vi "testRegEvtServersAandB.vi"(8 "error in (no error)":errorcluster) -> (0 "error out":errorcluster)   [LabVIEW 2018]
uses:
  src/FactoryTcpServer/FactoryTcpServer.lvclass
  src/TcpServer/TcpServer.lvclass/TcpServer.ctl
  src/TcpServerBase/TcpServerBase.lvclass/TcpServerBase.ctl
  src/TcpServerCmd/TcpServerCmd.lvclass
  home/pcortes/Documents/github/ts_labview_tcp_json/src/TcpServerBase/TcpServerBase.lvclass
  <vilib>/addons/_JKI Toolkits/Caraya/classes/Assert/Assert Equal Value_Variant.vi
  <vilib>/addons/_JKI Toolkits/Caraya/classes/Test/Test.lvclass
  <vilib>/addons/_JKI Toolkits/Caraya/classes/Assert/Assert.lvclass
  src/TcpServer/TcpServer.lvclass
  src/TcpServerBase/TcpServerBase.lvclass
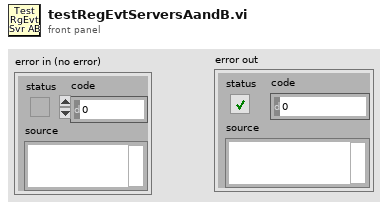
[diagram p1: front panel]
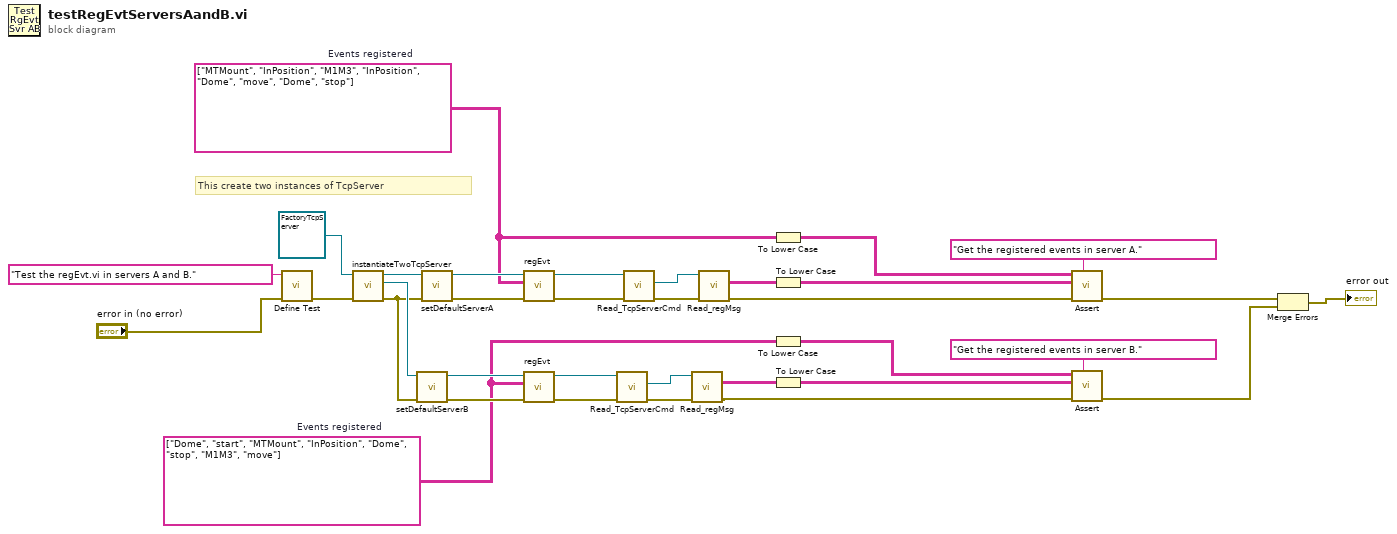
[diagram p0: block diagram]
diagram:
  w8 = string[][] [["Dome", "start"], ["MTMount", "InPosition"], ["Dome", "stop"], ["M1M3", "move"]]  # Events registered
  w13 = string[][] [["MTMount", "InPosition"], ["M1M3", "InPosition"], ["Dome", "move"], ["Dome", "stop"]]  # Events registered
  # "This create two instances of TcpServer"
  n1 = call <vilib>:"Define Test.vi"("error in (no error)"="error in (no error)", "Label (VI Title)"="Test the regEvt.vi in servers A and B.") -> ("error out"=w4:errorcluster)  [unwired: 9 in]
  n2 = call "instantiateTwoTcpServer.vi"("error in (no error)"=w4, "FactoryTcpServer in"=refnum<class "FactoryTcpServer.lvclass"> refnum) -> ("error out"=w1:errorcluster, "TcpServer 2 out"=w2:refnum<class "TcpServer.lvclass">, "TcpServer 1 out"=w3:refnum<class "TcpServer.lvclass">)  [unwired: 7 in]
  n3 = call "setDefaultServerB.vi"("error in (no error)"=w1, "TcpServer.lvclass"=w2) -> ("error out"=w28:errorcluster, "tcpServer out"=w27:refnum<class "TcpServer.lvclass">)  [unwired: 8 in]
  n4 = call "setDefaultServerA.vi"("error in (no error)"=w1, "TcpServer.lvclass"=w3) -> ("error out"=w30:errorcluster, "tcpServer out"=w29:refnum<class "TcpServer.lvclass">)  [unwired: 8 in]
  n5 = call "regEvt.vi"("error in (no error)"=w30, "evtReg"=w13, "tcpServer in"=w29) -> ("error out"=w19:errorcluster, "tcpServer out"=w18:refnum<class "TcpServer.lvclass">)  [unwired: 7 in]
  n6 = call "regEvt.vi"("error in (no error)"=w28, "evtReg"=w8, "tcpServer in"=w27) -> ("error out"=w16:errorcluster, "tcpServer out"=w17:refnum<class "TcpServer.lvclass">)  [unwired: 7 in]
  n7 = call "Read_TcpServerCmd.vi"("error in (no error)"=w16, "TcpServer in"=w17) -> ("error out"=w21:errorcluster, "TcpServerCmd.lvclass"=w20:refnum<class "TcpServerCmd.lvclass">)  [unwired: 7 in, 1 out]
  n8 = call "Read_TcpServerCmd.vi"("error in (no error)"=w19, "TcpServer in"=w18) -> ("error out"=w22:errorcluster, "TcpServerCmd.lvclass"=w23:refnum<class "TcpServerCmd.lvclass">)  [unwired: 7 in, 1 out]
  n9 = call "Read_regMsg.vi"("error in (no error)"=w21, "TcpServerBase in"=w20) -> ("error out"=w14:errorcluster, "regMsg"=w11:string[][])  [unwired: 7 in, 1 out]
  n10 = call "Read_regMsg.vi"("error in (no error)"=w22, "TcpServerBase in"=w23) -> ("error out"=w15:errorcluster, "regMsg"=w12:string[][])  [unwired: 7 in, 1 out]
  n11 = To Lower Case(string=w13) -> (all lower case string=w10:string[][])
  n12 = To Lower Case(string=w12) -> (all lower case string=w9:string[][])
  n13 = To Lower Case(string=w8) -> (all lower case string=w7:string[][])
  n14 = To Lower Case(string=w11) -> (all lower case string=w6:string[][])
  n15 = call-poly <vilib>:"Assert.vi"("Label"="Get the registered events in server A.", "error in (no error)"=w15, "Y"=w9, "X"=w10) -> ("error out"=w32:errorcluster)  [unwired: 7 in]
  n16 = call-poly <vilib>:"Assert.vi"("Label"="Get the registered events in server B.", "error in (no error)"=w14, "Y"=w6, "X"=w7) -> ("error out"=w24:errorcluster)  [unwired: 7 in]
  n17 = Merge Errors(w32, w24) -> (→"error out":errorcluster)
